vi "(Depricated) Sample Line Core.vi"(8 "error in (no error)":errorcluster, 11 "cRIO-CO2 in":refnum<class "cRIO-CO2.lvclass">) -> ()   [LabVIEW 2015, in "cRIO-Carbondioxide.lvlib" / "cRIO-CO2.lvlib" / "cRIO-CO2.lvclass"]
doc: "Reads Sample Line State variable. Opens a single line."
uses:
  cRIO-CO2.lvclass
  Controls/Sample Line State Enumerator.ctl
panel:
  out "Numeric":i32
  out "error out":errorcluster
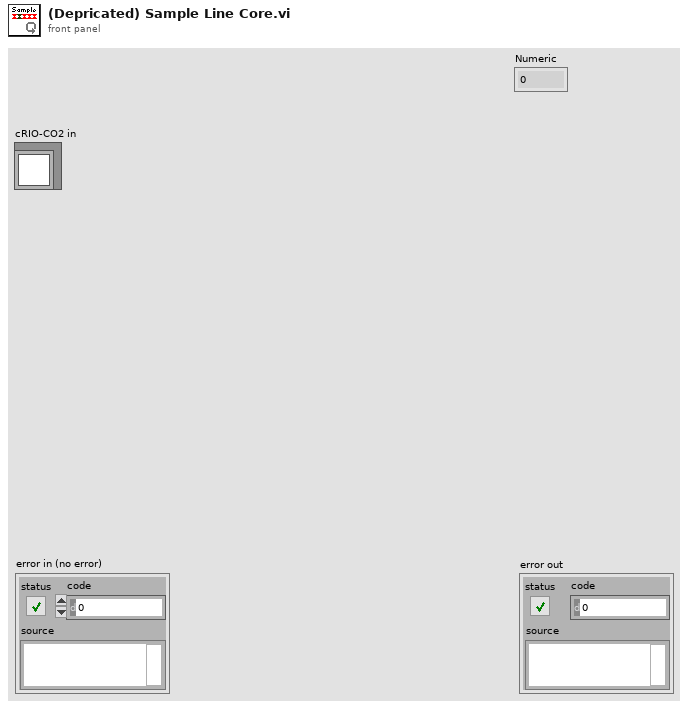
[diagram p1: front panel]
types:
  T1 = typedef "Sample Line State Enumerator.ctl" = enum16{"All lines closed", "Sample line 1.", "Sample line 2.", "Sample line 3.", "Sample line 4.", "Sample line 5.", "Out of range"}
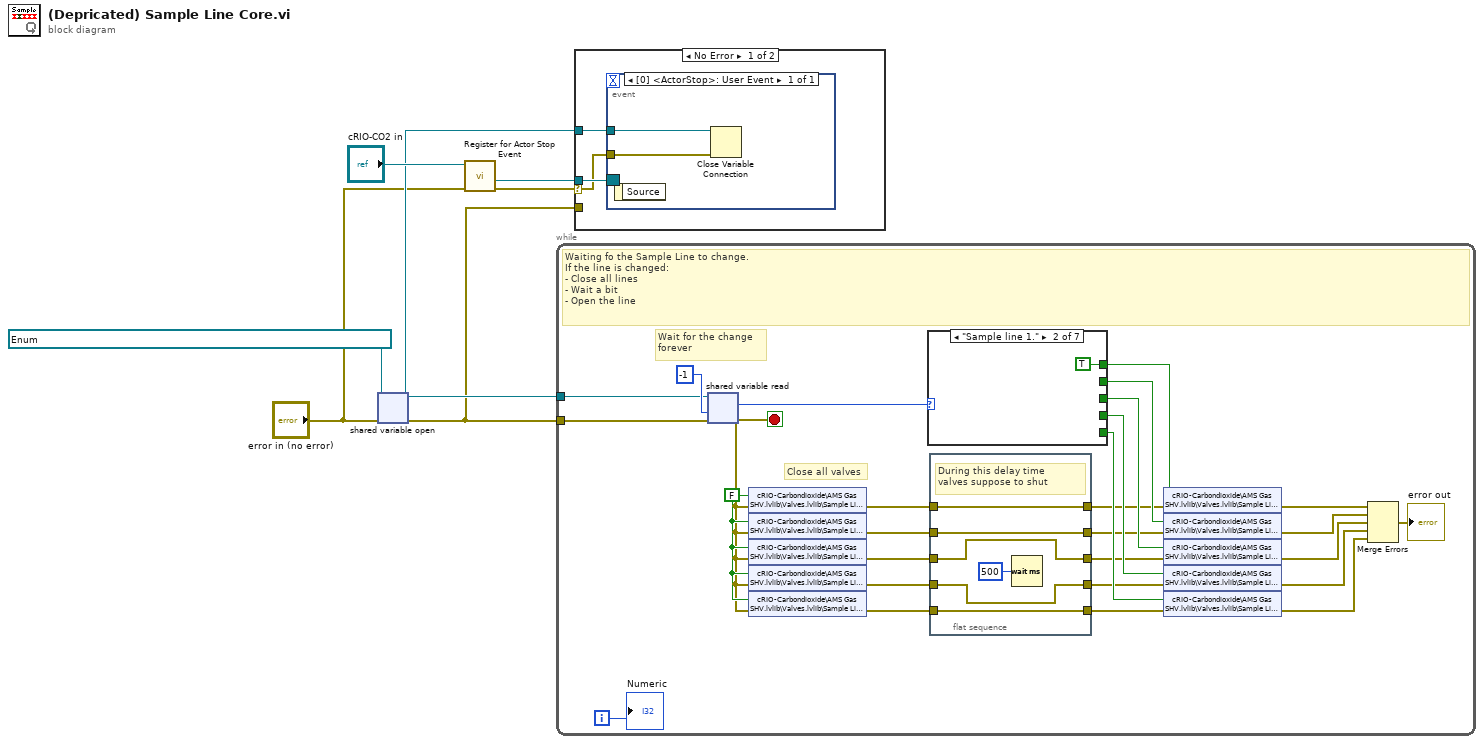
[diagram p0: block diagram]
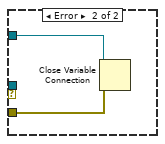
[diagram p2: hidden frame]
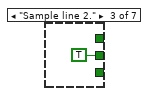
[diagram p4: hidden frame]
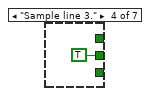
[diagram p5: hidden frame]
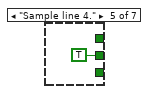
[diagram p6: hidden frame]
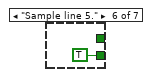
[diagram p7: hidden frame]
diagram:
  w4 = refnum<k21> "ni.var.psp://cRIO-Carbondioxide/AMS Gas SHV/Valves/Sample Line" items=["All lines closed", "Sample line 1.", "Sample line 2.", "Sample line 3.", "Sample line 4.", "Sample line 5.", "Out of range"] ("shared variable refnum in")
  n1 = shared-variable-open(w4, "error in (no error)") -> (w3:refnum<k21>, w1:errorcluster)
  n2 = call "Register for Actor Stop Event.vi"("error in (no error)"="error in (no error)", "cRIO-CO2 in"="cRIO-CO2 in") -> ("error out"=w6:errorcluster, "Event Registration Refnum"=w5:refnum<event-registration>)  [unwired: 7 in, 1 out]
  n3 = while {
    tunnel: w1 -> [w30]
    tunnel: w3 -> [w9]
    i -> [w10]
    stop <- w8 stop-if-true
    w28 = FALSE ("Sample Valve 1 DV314")
    # "Wait for the change \nforever"
    # "Close all valves"
    # "Waiting fo the Sample Line to change.\nIf the line is changed:\n- Close all lines\n- Wait a bit\n- Open the line"
    n4 = shared-variable-read(w9, w30, -1 ("ms timeout (0)")) -> (w8:errorcluster, w27:T1)  [unwired: 2 out]
    n5 = shared-variable "cRIO-Carbondioxide\\AMS Gas SHV.lvlib\\Valves.lvlib\\Sample Line Valves.lvlib\\Sample Line 1"(w28, error in=w8) -> (error out=w20:errorcluster)
    n6 = shared-variable "cRIO-Carbondioxide\\AMS Gas SHV.lvlib\\Valves.lvlib\\Sample Line Valves.lvlib\\Sample Line 2"(w28, error in=w8) -> (error out=w18:errorcluster)
    n7 = shared-variable "cRIO-Carbondioxide\\AMS Gas SHV.lvlib\\Valves.lvlib\\Sample Line Valves.lvlib\\Sample Line 3"(w28, error in=w8) -> (error out=w16:errorcluster)
    n8 = shared-variable "cRIO-Carbondioxide\\AMS Gas SHV.lvlib\\Valves.lvlib\\Sample Line Valves.lvlib\\Sample Line 4"(w28, error in=w8) -> (error out=w14:errorcluster)
    n9 = shared-variable "cRIO-Carbondioxide\\AMS Gas SHV.lvlib\\Valves.lvlib\\Sample Line Valves.lvlib\\Sample Line 5"(w28, error in=w8) -> (error out=w12:errorcluster)
    n10 = case shown="\"Sample line 1.\"" w27 {
      tunnel: [_ TRUE _ _ _ _ _] -> w26
      tunnel: [_ _ TRUE _ _ _ _] -> w23
      tunnel: [_ _ _ TRUE _ _ _] -> w22
      tunnel: [_ _ _ _ TRUE _ _] -> w25
      tunnel: [_ _ _ _ _ TRUE _] -> w24
      frame "All lines closed", Default {
      }
      frame "Sample line 1." {
      }
      frame "Sample line 2." {
      }
      frame "Sample line 3." {
      }
      frame "Sample line 4." {
      }
      frame "Sample line 5." {
      }
      frame "Out of range" {
        # "Value is out of range.\nClose all valves"
      }
    }
    n11 = flat-sequence {
      tunnel: w20 -> [w41]
      tunnel: [w41] -> w19
      tunnel: w18 -> [w40]
      tunnel: [w40] -> w17
      tunnel: w16 -> [w38]
      tunnel: [w38] -> w15
      tunnel: w14 -> [w37]
      tunnel: [w37] -> w13
      tunnel: w12 -> [w39]
      tunnel: [w39] -> w11
      frame #0 {
        # "During this delay time\nvalves suppose to shut"
        n12 = Wait (ms)(milliseconds to wait=u32 500) -> ()  [unwired: 1 out]
      }
    }
    n13 = shared-variable "cRIO-Carbondioxide\\AMS Gas SHV.lvlib\\Valves.lvlib\\Sample Line Valves.lvlib\\Sample Line 1"(w26, error in=w19) -> (error out=w35:errorcluster)
    n14 = shared-variable "cRIO-Carbondioxide\\AMS Gas SHV.lvlib\\Valves.lvlib\\Sample Line Valves.lvlib\\Sample Line 2"(w23, error in=w17) -> (error out=w34:errorcluster)
    n15 = shared-variable "cRIO-Carbondioxide\\AMS Gas SHV.lvlib\\Valves.lvlib\\Sample Line Valves.lvlib\\Sample Line 3"(w22, error in=w15) -> (error out=w33:errorcluster)
    n16 = shared-variable "cRIO-Carbondioxide\\AMS Gas SHV.lvlib\\Valves.lvlib\\Sample Line Valves.lvlib\\Sample Line 4"(w25, error in=w13) -> (error out=w29:errorcluster)
    n17 = shared-variable "cRIO-Carbondioxide\\AMS Gas SHV.lvlib\\Valves.lvlib\\Sample Line Valves.lvlib\\Sample Line 5"(w24, error in=w11) -> (error out=w32:errorcluster)
    n18 = Merge Errors(w35, w34, w33, w29, w32) -> (→"error out":errorcluster)
    "Numeric" <- w10
  }
  n19 = case shown="No Error" w6 {
    selector: w6 -> [w47 _]
    tunnel: w5 -> [w49 _]
    tunnel: w3 -> [w48 w53]
    tunnel: w1 -> [_ w52]
    frame No Error {
      n20 = event shown="[0] <ActorStop>: User Event" {
        selector: w49 -> [_]
        dyn-events: _ -> [_]
        timeout: _ -> [_]
        tunnel: w48 -> [w51]
        tunnel: w47 -> [w50]
        event User Event {
          n21 = event-data() -> ()  [unwired: 1 in, 1 out]
          n22 = Close Variable Connection(8:w50, 11:w51) -> ()  [unwired: 1 out]
        }
      }
    }
    frame Error {
      n23 = Close Variable Connection(8:w52, 11:w53) -> ()  [unwired: 1 out]
    }
  }
